vi "Read User Name.vi"(6 "User group":u16, 9 "Pass word":string, 10 "用户登录":T1, 11 "User name":string) -> (2 "Pass fail":bool, 3 "User fail":bool)   [LabVIEW 2017]
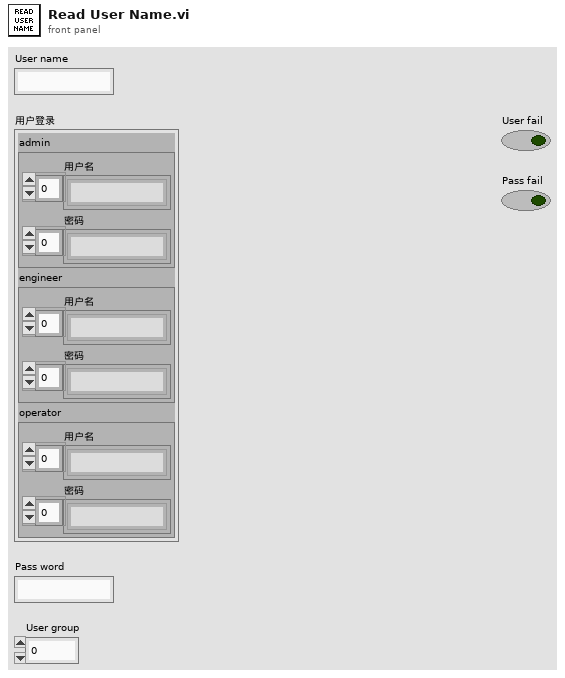
[diagram p1: front panel]
types:
  T1 = cluster{"admin":cluster{"用户名":string[], "密码":string[]}, "engineer":cluster{"用户名":string[], "密码":string[]}, "operator":cluster{"用户名":string[], "密码":string[]}}
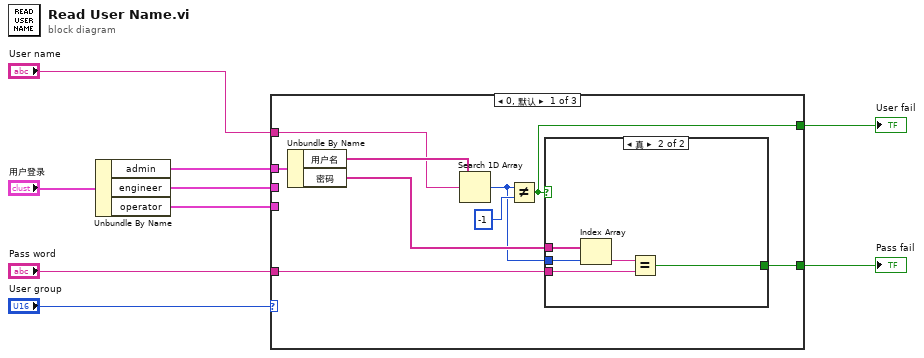
[diagram p0: block diagram]
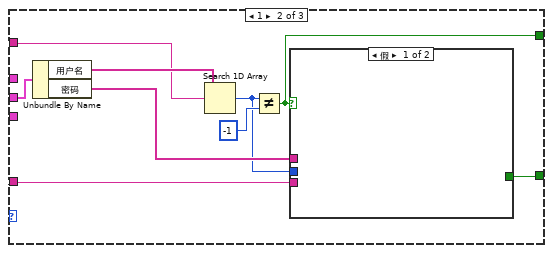
[diagram p3: hidden frame]
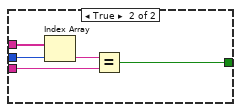
[diagram p4: hidden frame]
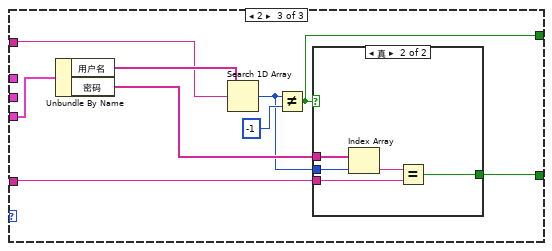
[diagram p5: hidden frame]
diagram:
  n1 = Unbundle By Name("用户登录") -> ("admin"=w3:cluster{"用户名":string[], "密码":string[]}, "engineer"=w4:cluster{"用户名":string[], "密码":string[]}, "operator"=w5:cluster{"用户名":string[], "密码":string[]})
  n2 = case shown="0, 默认" "User group" {
    tunnel: w3 -> [w18 _ _]
    tunnel: w4 -> [_ w24 _]
    tunnel: w5 -> [_ _ w41]
    tunnel: "User name" -> [w15 w28 w42]
    tunnel: "Pass word" -> [w12 w27 w40]
    tunnel: [w11 w26 w39] -> w8
    tunnel: [w10 w25 w38] -> w9
    frame 0, Default {
      n3 = Unbundle By Name(w18) -> ("用户名"=w17:string[], "密码"=w14:string[])
      n4 = Search 1D Array(1D array=w17, element=w15) -> (index of element=w13:i32)  [unwired: 1 in]
      n5 = Not Equal?(x=w13, y=-1) -> (x != y?=w10:bool)
      n6 = case shown="真" w10 {
        tunnel: w14 -> [_ w23]
        tunnel: w13 -> [_ w22]
        tunnel: w12 -> [_ w20]
        tunnel: [_ w19] -> w11
        frame False {
        }
        frame True {
          n7 = Index Array(array=w23, index=w22) -> (element=w21:string)
          n8 = Equal?(x=w21, y=w20) -> (x = y?=w19:bool)
        }
      }
    }
    frame 1 {
      n9 = Unbundle By Name(w24) -> ("用户名"=w32:string[], "密码"=w30:string[])
      n10 = Search 1D Array(1D array=w32, element=w28) -> (index of element=w29:i32)  [unwired: 1 in]
      n11 = Not Equal?(x=w29, y=-1) -> (x != y?=w25:bool)
      n12 = case shown="假" w25 {
        tunnel: w30 -> [_ w37]
        tunnel: w29 -> [_ w36]
        tunnel: w27 -> [_ w34]
        tunnel: [_ w33] -> w26
        frame False {
        }
        frame True {
          n13 = Index Array(array=w37, index=w36) -> (element=w35:string)
          n14 = Equal?(x=w35, y=w34) -> (x = y?=w33:bool)
        }
      }
    }
    frame 2 {
      n15 = Unbundle By Name(w41) -> ("用户名"=w46:string[], "密码"=w44:string[])
      n16 = Search 1D Array(1D array=w46, element=w42) -> (index of element=w43:i32)  [unwired: 1 in]
      n17 = Not Equal?(x=w43, y=-1) -> (x != y?=w38:bool)
      n18 = case shown="真" w38 {
        tunnel: w44 -> [_ w51]
        tunnel: w43 -> [_ w50]
        tunnel: w40 -> [_ w48]
        tunnel: [_ w47] -> w39
        frame False {
        }
        frame True {
          n19 = Index Array(array=w51, index=w50) -> (element=w49:string)
          n20 = Equal?(x=w49, y=w48) -> (x = y?=w47:bool)
        }
      }
    }
  }
  "Pass fail" <- w8
  "User fail" <- w9
